vi "Units_RadiansToDegrees.vi"(10 "Radians":dbl) -> (2 "Degrees":dbl)   [LabVIEW 2019, in "Trajectory_Library.lvlib"]
doc: "Convert a angle value from radians to degrees\n\nInputs: \n - Radians - Angle (Radians)\n\nOutputs:\n - Degrees - Angle (Degrees)"
uses:
  Trajectory_Library.lvlib
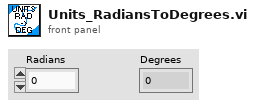
[diagram p1: front panel]
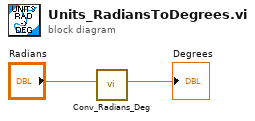
[diagram p0: block diagram]
diagram:
  n1 = call "Conv_Radians_Deg.vi"("Radians"="Radians") -> ("Degrees"=→"Degrees":dbl)  [unwired: 10 in]
